vi "Constructor.vi"(8 "error in":errorcluster, 11 "Main Path":path) -> (0 "error out":errorcluster)   [LabVIEW 2012, in "Error Logger.lvclass"]
uses:
  Error Logger.lvclass
  Error Logger.lvclass/Error Logger.ctl
  Write File Ref.vi
  Write Current File Path.vi
  Write Main Path.vi
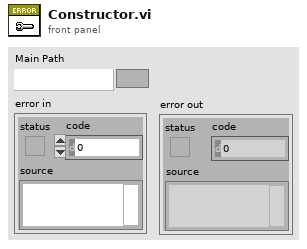
[diagram p1: front panel]
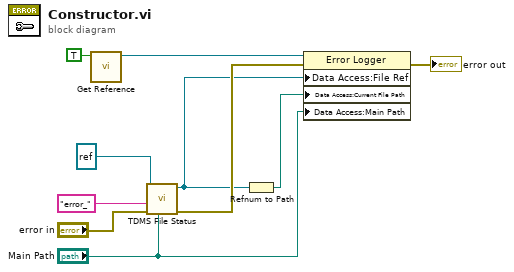
[diagram p0: block diagram]
diagram:
  n1 = call "Get Reference.vi"("Init?"=TRUE) -> ("DVR"=w9:refnum<data-value>)  [unwired: 9 in, 1 out]
  n2 = call "TDMS File Status.vi"("Data Path"="Main Path", "erriorIn"="error in", "prefix"="error_", "fileRefIn"=refnum<k34> refnum) -> ("error out"=w5:errorcluster, "tdms file out"=w3:refnum<k34>)  [unwired: 6 in]
  n3 = Refnum to Path(1:w3) -> (0:w2:path)
  n4 = property class="Error Logger"(reference=w9, error in=w5, "Data Access:File Ref"=w3, "Data Access:Current File Path"=w2, "Data Access:Main Path"="Main Path") -> (error out=→"error out":errorcluster)  [unwired: 1 out]
